vi "manda_json_firebase.vi"() -> ()   [LabVIEW 2025]
uses:
  <vilib>/httpClient/PUTBuffer.vi
  <vilib>/httpClient/LabVIEWHTTPClient.lvlib
panel:
  in  "Nombre":string
  in  "Apeido":string
  out "headers":string
  out "body":string
  out "error out":errorcluster
  in  "stop":bool
  in  "Edad":dbl
  in  "Rele":bool
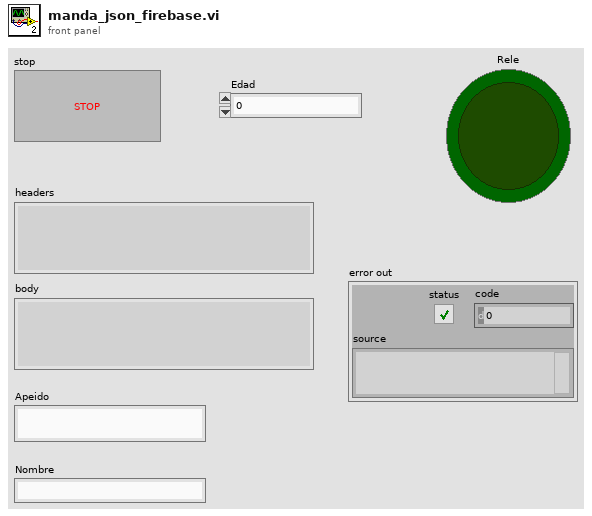
[diagram p1: front panel]
types:
  T1 = cluster{"Apeido":string, "Edad":dbl, "Fecha":string, "Hora":string, "Nombre":string, "Rele":bool}
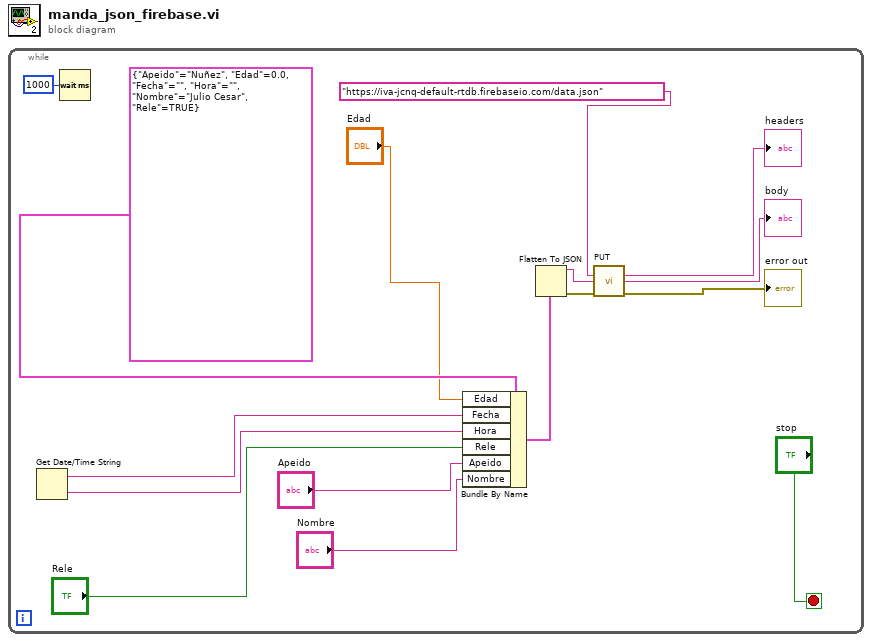
[diagram p0: block diagram]
diagram:
  n1 = while {
    stop <- "stop" stop-if-true
    n2 = Get Date/Time String() -> (date string=w4:string, time string=w3:string)  [unwired: 3 in]
    n3 = Wait (ms)(milliseconds to wait=u32 1000) -> ()  [unwired: 1 out]
    n4 = Bundle By Name(cluster=T1 {"Apeido"="Nuñez", "Edad"=0.0, "Fecha"="", "Hora"="", "Nombre"="Julio Cesar", "Rele"=TRUE}, "Edad"="Edad", "Fecha"=w4, "Hora"=w3, "Rele"="Rele", "Apeido"="Apeido", "Nombre"="Nombre") -> (w10:T1)
    n5 = Flatten To JSON(anything=w10) -> (JSON string=w9:string, 11:w8:errorcluster)  [unwired: 2 in]
    n6 = call-poly <vilib>:"PUT.vi"("url"="https://iva-jcnq-default-rtdb.firebaseio.com/data.json", "buffer"=w9, "error in (no error)"=w8) -> ("headers"=→"headers":string, "body"=→"body":string, "error out"=→"error out":errorcluster)  [unwired: 9 in, 1 out]
  }
